vi "GetPersistentConfiguration.vi"(8 "ErrorIn":errorcluster, 9 "DataIn":variant, 11 "ObjectIn":refnum<class "IPersistentData.lvclass">) -> (0 "ErrorOut":errorcluster, 1 "DataOut":variant, 3 "ObjectOut":refnum<class "IPersistentData.lvclass">)   [LabVIEW 2021, in "IPersistentData.lvclass"]
uses:
  IPersistentData.lvclass
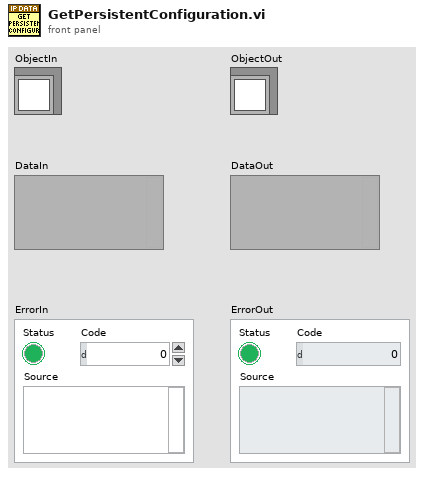
[diagram p1: front panel]
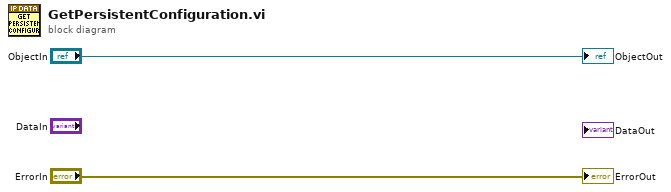
[diagram p0: block diagram]
diagram:
  "ErrorOut" <- "ErrorIn"
  "ObjectOut" <- "ObjectIn"
